vi "YoutuberDownloader.vi"(8 "error in (no error)":errorcluster, 10 "ThirdPartyYoutubeLib.lvclass":refnum<class "ThirdPartyYoutubeLib.lvclass">, 11 "YoutuberDownloader in":refnum<class "YoutuberDownloader.lvclass">) -> (0 "error out":errorcluster, 3 "YoutuberDownloader out":refnum<class "YoutuberDownloader.lvclass">)   [LabVIEW 2018, in "YoutuberDownloader.lvclass"]
uses:
  YoutuberDownloader.lvclass
  ThirdPartyYoutubeLib Class/ThirdPartyYoutubeLib.lvclass
  YoutuberDownloader.lvclass/YoutuberDownloader.ctl
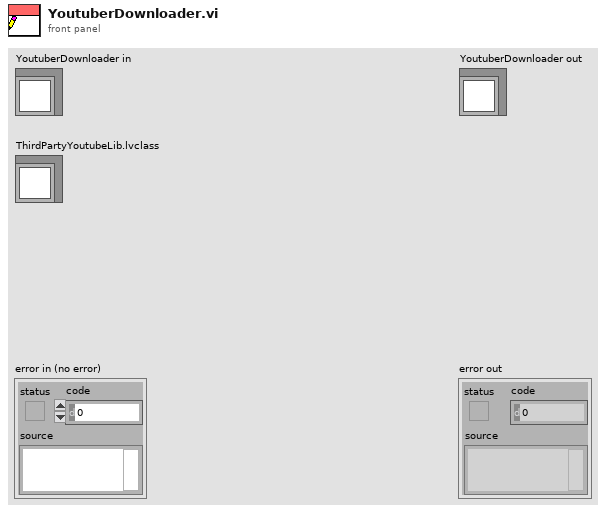
[diagram p1: front panel]
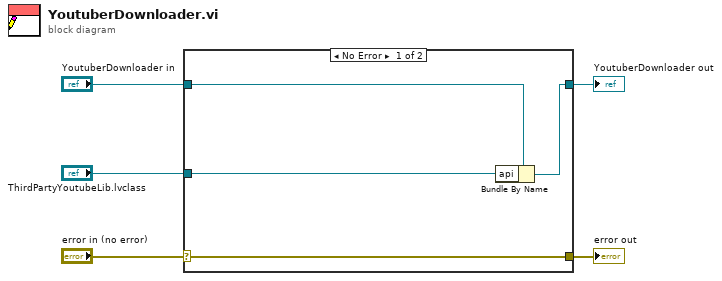
[diagram p0: block diagram]
diagram:
  n1 = case shown="No Error" "error in (no error)" {
    selector: "error in (no error)" -> [w9 w10]
    tunnel: [w9 w10] -> w4
    tunnel: [w7 w11] -> w2
    tunnel: "YoutuberDownloader in" -> [w8 w11]
    tunnel: "ThirdPartyYoutubeLib.lvclass" -> [w6 _]
    frame No Error {
      n2 = Bundle By Name(cluster=w8, "api"=w6) -> (w7:refnum<class "YoutuberDownloader.lvclass">)
    }
    frame Error {
    }
  }
  "error out" <- w4
  "YoutuberDownloader out" <- w2
